vi "LUT.vi"(11 "Hub Distance (ft)":dbl) -> (2 "Hood Setpoint":dbl, 3 "Shooter RPM":dbl)   [LabVIEW 2025]
panel:
  out "Fractional Index":dbl
  out "Step Size":i32
  out "Start Distance":i32
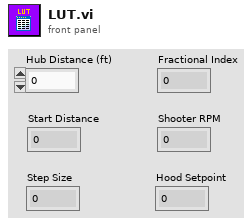
[diagram p1: front panel]
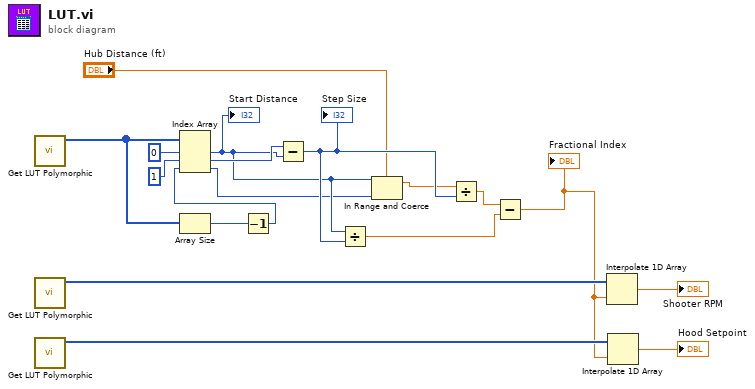
[diagram p0: block diagram]
diagram:
  n1 = call-poly "Get LUT Polymorphic.vi"() -> ("LUT Out"=w11:i32[])  [unwired: 10 in, 1 out]
  n2 = call-poly "Get LUT Polymorphic.vi"() -> ("LUT Out"=w10:i32[])  [unwired: 10 in, 1 out]
  n3 = call-poly "Get LUT Polymorphic.vi"() -> ("LUT Out"=w9:i32[])  [unwired: 10 in, 1 out]
  n4 = Array Size(array=w11) -> (size(s)=w15:i32)
  n5 = Decrement(x=w15) -> (x-1=w14:i32)
  n6 = Index Array(array=w11, index #1=0 ("index"), index #2=1 ("index"), index #3=w14) -> (element #1=w2:i32, element #2=w16:i32, element #3=w1:i32)
  "Start Distance" <- w2
  n7 = Subtract(x=w16, y=w2) -> (x-y=w6:i32)
  "Step Size" <- w6
  n8 = Divide(x=w2, y=w6) -> (x/y=w5:dbl)
  n9 = In Range and Coerce(upper limit=w2, x="Hub Distance (ft)", lower limit=w1) -> (coerced(x)=w3:dbl)  [unwired: 1 out]
  n10 = Divide(x=w3, y=w6) -> (x/y=w8:dbl)
  n11 = Subtract(x=w8, y=w5) -> (x-y=w7:dbl)
  "Fractional Index" <- w7
  n12 = Interpolate 1D Array(1:w7, 2:w10) -> (0:→"Shooter RPM":dbl)
  n13 = Interpolate 1D Array(1:w7, 2:w9) -> (0:→"Hood Setpoint":dbl)
